vi "Main.vi"() -> ()   [LabVIEW 2012]
uses:
  <vilib>/Platform/TimedLoop/XDataNode/timing_clust.ctl
  <vilib>/Platform/TimedLoop/XDataNode/nitl_modes.ctl
  <vilib>/Platform/TimedLoop/XDataNode/wakeup.ctl
  Sensors and Mapping/Global_grid settings.vi
  <vilib>/FPGAPlugInAG/sbRIO-9636/niLvFpga_Open_sbRIO-9636.vi
  <vilib>/rvi/interface/common/dynamic/niFpgaDynamicAddResources.vi
  <vilib>/Utility/error.llb/Error Cluster From Error Code.vi
  <vilib>/rvi/errors/niLvFpgaAdjustHostInterfaceError.vi
  <vilib>/Analysis/coordinate.llb/2D Cartesian Coordinate Rotation (Scalar).vi
  <vilib>/FPGAPlugInAG/Dynamic/niLvFpga_Close_Dynamic.vi
  <vilib>/Platform/TimedLoop/XDataNode/XDataNode.xnode
  <vilib>/rvi/interface/nirviOpenFPGA/nirviOpenFPGA.xnode
  FPGA Bitfiles/NIARCDemo-kyle_FPGATarget_FPGAToplevel_9c4As6+H2cU.lvbitx
  <vilib>/rvi/interface/nirviReadWriteControl/nirviReadWriteControl.xnode
  <vilib>/robotics/Navigation/shared/WorldMap/OccupancyGridWorldMap/NI_Robotics_OccupancyGridWorldMap.lvclass
  <vilib>/rvi/interface/nirviCloseFPGA/nirviCloseFPGA.xnode
  <vilib>/Platform/TimedLoop/XDataNode/XDNodeRunTimeDep.lvlib
  Compass/Compass IO.lvlib
  Mouse IO/Mouse IO.lvlib
  <vilib>/Analysis/NI_AALPro.lvlib
  NiFpgaLv.dll
  <vilib>/rvi/interface/Simulation/niFpgaSimulationCallBeginRW.vi
panel:
  in  "Max Distance":dbl=0.8
  in  "Robot Velocities":T1 {"Angular Velocity (rad/s)" min=-1.0 max=1.0 scale=1.0..-1.0; "Y Velocity (m/s)" min=-1.0 max=1.0 scale=-1.0..1.0; "X Velocity (m/s)" min=-1.0 max=1.0 scale=-1.0..1.0}
  in  "Enable":bool
  out "Robot Location":cluster{"X array":dbl[], "Y array":dbl[]}(graph)
  out "Robot y":dbl
  out "Robot x":dbl
  out "Heading (deg)":dbl
  out "Object Array":cluster{"Sensor X":dbl, "Sensor Y":dbl}[](array[cluster])
  out "Sensor Distances":fxp<+/-,26,5>[](array[numeric])
  out "Iteration Duration":i64
  out "Sensor position Global":cluster{"Object X":dbl, "Object Y":dbl}
  in  "Robot position Global":T2 {"Orientation (rad)" step=0.1}
  out "Finished late":bool
  out "Object Map":dbl[][](graph)
  in  "x start":i32
  in  "y start":i32
  in  "stop":bool
  # "Goal"
  # "Start"
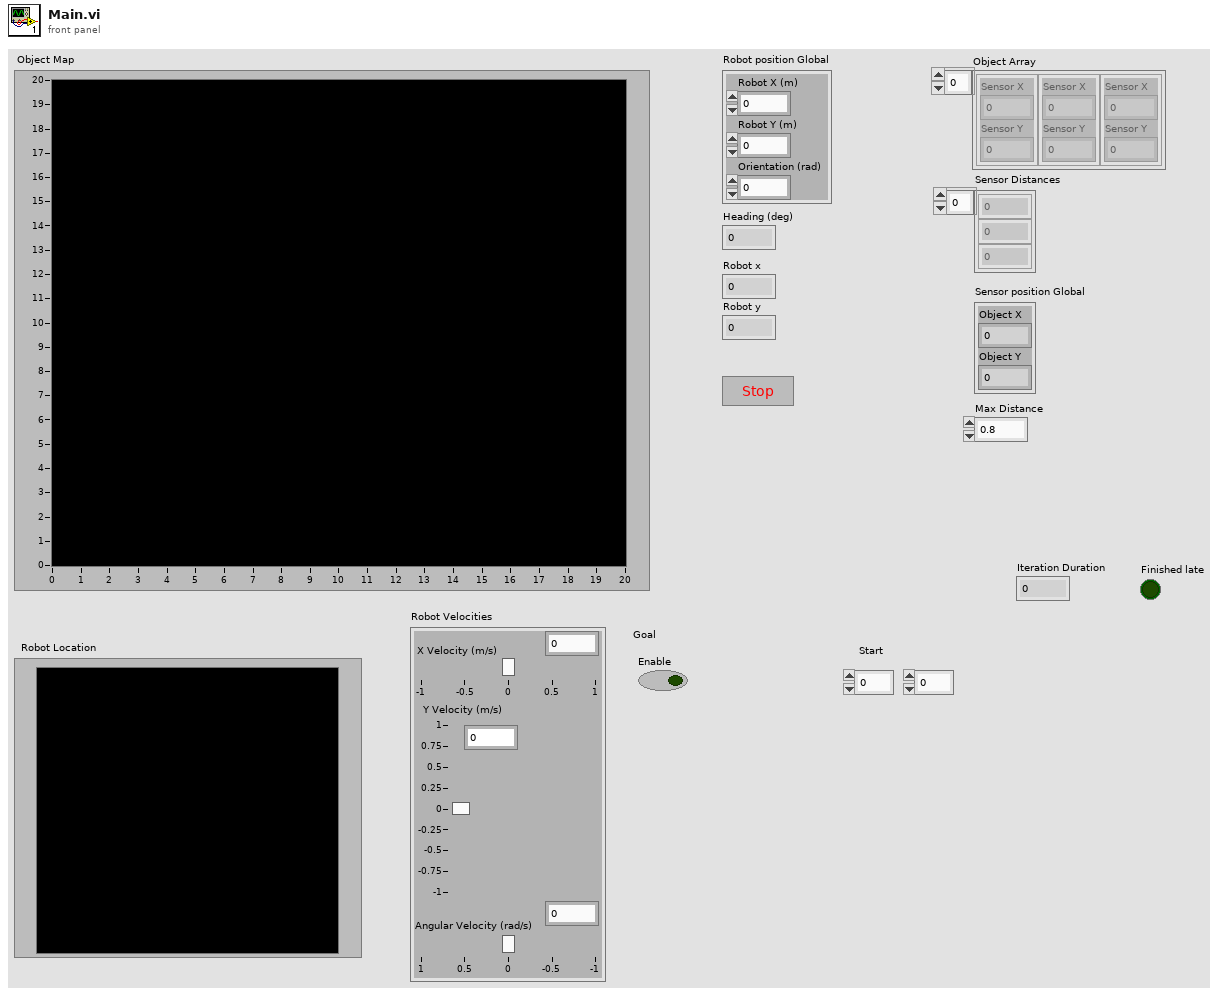
[diagram p1: front panel]
types:
  T1 = cluster{"X Velocity (m/s)":dbl, "Y Velocity (m/s)":dbl, "Angular Velocity (rad/s)":dbl}
  T2 = cluster{"Robot X (m)":dbl, "Robot Y (m)":dbl, "Orientation (rad)":dbl}
  T3 = cluster{"sensor x":dbl, "sensor y":dbl, "sensor rot (rad)":dbl}[]
  T4 = cluster{"X cells":i32, "Y cells":i32, "X size (m)":dbl, "Y size (m)":dbl}
  T5 = cluster{"FPGA VI Reference":refnum<k20>, "Timeout":i32}
  T6 = cluster{"FPGA VI Reference":refnum<k20>, "Port Number":u8}
  T7 = typedef "XDNodeRunTimeDep.lvlib/timing_clust.ctl" = cluster{"Expected End [f-1]":u64, "Actual End [f-1]":u64, "Finished Late? [f-1]":bool, "Expected End [i-1]":u64, "Actual End [i-1]":u64, "Finished Late? [i-1]":bool, "Expected Start [i]":u64, "Actual Start [i]":u64, "Expected Start [f]":u64, "Actual Start [f]":u64, "Source Name":string, "Structure Name":string, "Period":i64, "Deadline":i64, "Offset":i64, "Start":i64, "Priority":i32, "Timeout":i32, "Mode":T8, "Wakeup Reason":T9, "Error":errorcluster, "Source Type":string, "Secondary Source Type":string, "Global End Time":u64, "Global Start Time":u64, "Frame Duration":u64, "Iteration Duration":u64, "Assigned CPU":i32, "I/O Scan Engine Mode":u32}
  T8 = typedef "XDNodeRunTimeDep.lvlib/nitl_modes.ctl" = enum32{"No Change", "Process missed periods, maintain original phase", "Discard missed periods, maintain original phase", "Process missed periods, ignore original phase", "Discard missed periods, ignore original phase"}
  T9 = typedef "XDNodeRunTimeDep.lvlib/wakeup.ctl" = enum32{"Normal", "Aborted", "Asynchronous wakeup", "Timing source error", "Timed loop error", "Timeout"}
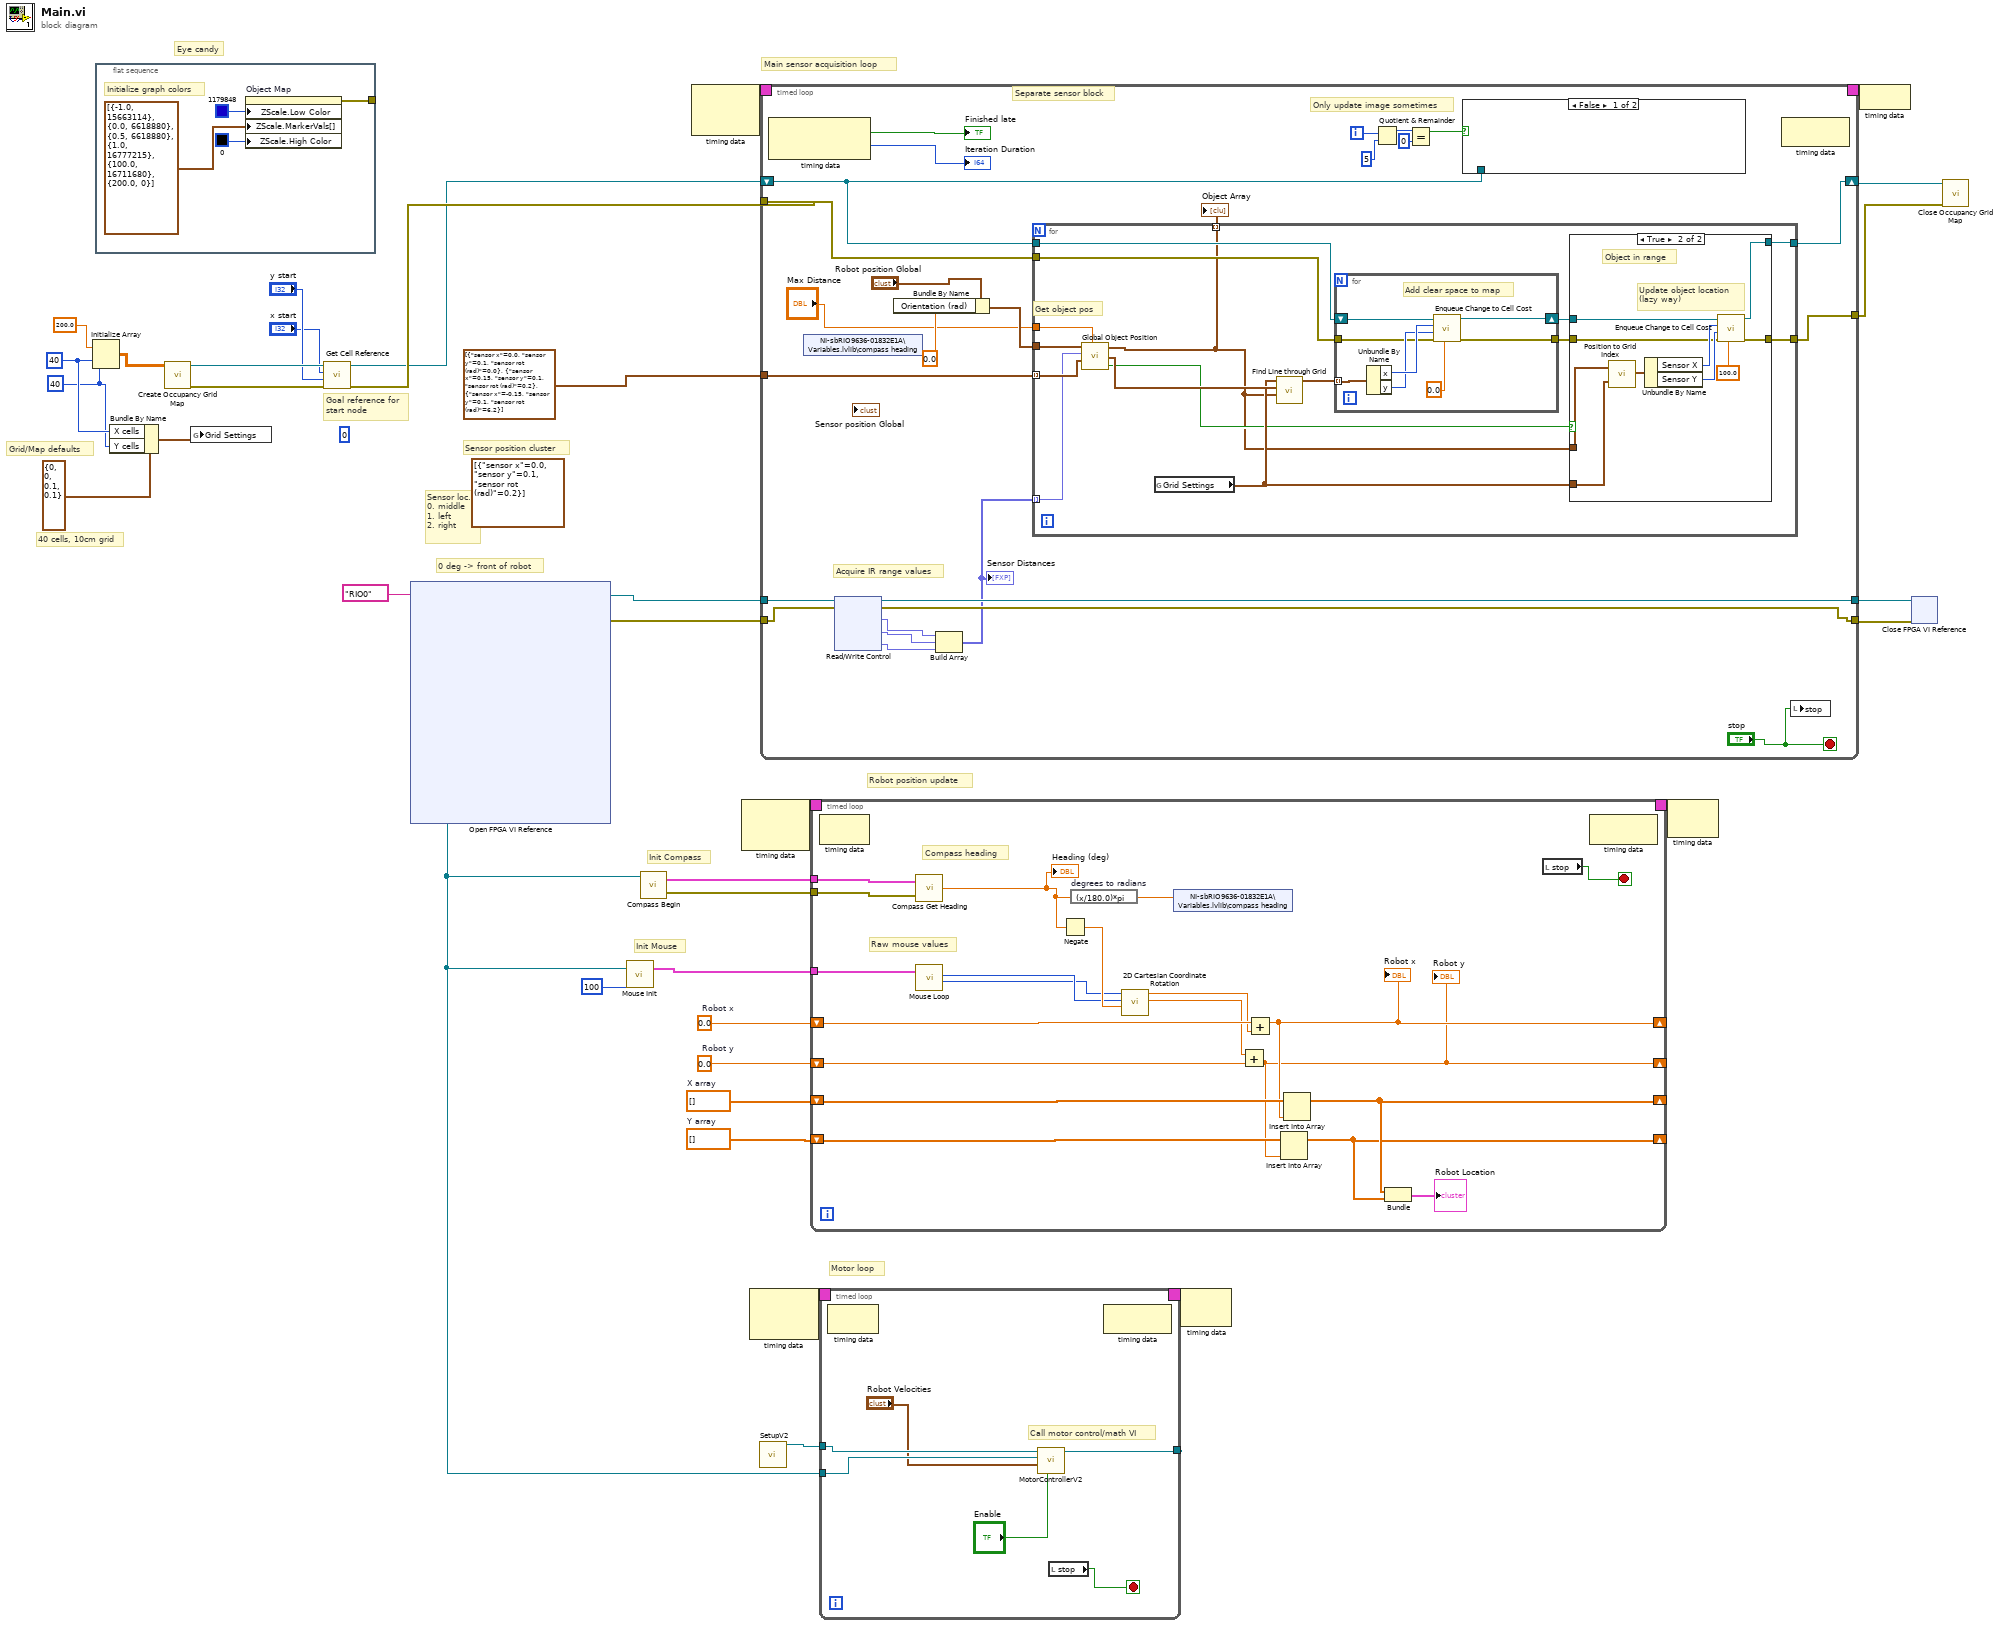
[diagram p0: block diagram]
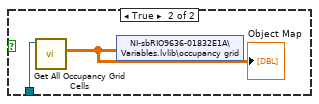
[diagram p3: hidden frame]
diagram:
  w5 = dbl[] []  # Y array
  w6 = dbl[] []  # X array
  w9 = 0.0  # Robot y
  w10 = 0.0  # Robot x
  (unwired) T3 [{"sensor x"=0.0, "sensor y"=0.1, "sensor rot (rad)"=0.0}, {"sensor x"=0.15, "sensor y"=0.1, "sensor rot (rad)"=0.2}, {"sensor x"=-0.15, "sensor y"=0.1, "sensor rot (rad)"=6.2}]
  (unwired) T3 [{"sensor x"=0.0, "sensor y"=0.1, "sensor rot (rad)"=0.2}]
  w24 = 40 ("dimension size")
  w25 = 40 ("dimension size")
  (unwired) 0
  # "Motor loop"
  # "Init Mouse"
  # "Init Compass"
  # "Robot position update"
  # "Main sensor acquisition loop"
  # "Sensor loc.:\n0. middle\n1. left\n2. right"
  # "Sensor position cluster"
  # "Eye candy"
  # "40 cells, 10cm grid"
  # "Grid/Map defaults"
  # "0 deg -> front of robot"
  # "Separate sensor block"
  # "Goal reference for\nstart node"
  n1 = Initialize Array(200.0 ("element"), w25, w24) -> (w29:dbl[][])
  n2 = flat-sequence {
    tunnel: [w36] -> _
    frame #0 {
      # "Initialize graph colors"
      n3 = property on="Object Map" class="IntGraph (strict)"("ZScale.Low Color"=u32 1179848, "ZScale.MarkerVals[]"=cluster{dbl, u32}[] [{-1.0, 15663114}, {0.0, 6618880}, {0.5, 6618880}, {1.0, 16777215}, {100.0, 16711680}, {200.0, 0}], "ZScale.High Color"=u32 0) -> (error out=w36:errorcluster)  [unwired: 2 in, 1 out]
    }
  }
  n4 = Bundle By Name(cluster=T4 {"X cells"=0, "Y cells"=0, "X size (m)"=0.1, "Y size (m)"=0.1} ("Grid Settings"), "X cells"=w25, "Y cells"=w24) -> (w27:T4)
  n5 = call <vilib>:"Create Occupancy Grid Map.vi"("occupancy grid"=w29) -> ("error out"=w32:errorcluster, "map reference out"=w33:refnum<data-value>)  [unwired: 9 in]
  n6 = global write "Global_grid settings.vi" "Grid Settings"(w27) -> ()
  n7 = call <vilib>:"Get Cell Reference.vi"("error in (no error)"=w32, "y"="y start", "x"="x start", "map reference in"=w33) -> ("error out"=w23:errorcluster, "map reference out"=w16:refnum<data-value>)  [unwired: 4 in, 2 out]
  n8 = xnode "Open FPGA VI Reference"("resource name"=tag "RIO0") -> ("FPGA VI Reference Out"=w1:refnum<k20>, "error out"=w20:errorcluster)  [unwired: 1 in]
  n9 = call "Mouse Init.vi"("Timeout (ms)"=100, "FPGA VI Reference In"=w1) -> ("Mouse Sensor"=w11:T5)  [unwired: 1 out]
  n10 = call "Compass Begin.vi"("FPGA VI Reference"=w1) -> ("error out"=w7:errorcluster, "FPGA Information Out"=w8:T6)  [unwired: 3 in]
  n11 = node-c288() -> (w35:T7)  [unwired: 2 in]
  n12 = node-c288() -> (w13:T7)  [unwired: 2 in]
  n13 = node-c288() -> (w4:T7)  [unwired: 2 in]
  n14 = call "SetupV2.vi"() -> ("mecanum steering frame out"=w2:refnum<class "NI_Robotics_Mecanum Steering Frame.lvclass">)  [unwired: 10 in, 1 out]
  n15 = timed-loop {
    timing: w35 -> [_]
    timing-out: [_] -> w34
    shift-right: [w58] -> w22
    shift-left: w16 -> [w51]
    tunnel: [w57] -> w21
    tunnel: w23 -> [w56]
    tunnel: T3 [{"sensor x"=0.0, "sensor y"=0.1, "sensor rot (rad)"=0.0}, {"sensor x"=-0.15, "sensor y"=0.1, "sensor rot (rad)"=0.0872664625997165}, {"sensor x"=0.15, "sensor y"=0.1, "sensor rot (rad)"=6.19591884457987}] -> [w47]
    tunnel: [w49] -> w19
    tunnel: w1 -> [w55]
    tunnel: [w48] -> w18
    tunnel: w20 -> [w54]
    i -> [w63]
    stop <- "stop" stop-if-true
    # "Acquire IR range values"
    # "Only update image sometimes"
    n16 = node-c288() -> (→"Finished late":bool, →"Iteration Duration":i64)  [unwired: 1 in]
    n17 = shared-variable "NI-sbRIO9636-01832E1A\\Variables.lvlib\\compass heading"() -> ()  [unwired: 1 in, 2 out]
    n18 = xnode "Read/Write Control"("FPGA VI Reference In"=w55, "error in"=w54) -> ("FPGA VI Reference Out"=w49:refnum<k20>, "error out"=w48:errorcluster, "IR 0"=w53:fxp<+/-,24,5>, "IR 2"=w50:fxp<+/-,24,5>, "IR 3"=w52:fxp<+/-,24,5>)
    n19 = Bundle By Name(cluster="Robot position Global", "Orientation (rad)"=0.0 ("compass heading")) -> (w42:T2)
    n20 = Build Array(w53, w50, w52) -> (w46:fxp<+/-,24,5>[])
    "Sensor Distances" <- w46
    n21 = for {
      tunnel: w42 -> [w80]
      tunnel: [w79] -> w58
      tunnel: [w78] -> w57
      tunnel: w56 -> [w77]
      tunnel: "Max Distance" -> [w76]
      tunnel: w51 -> [w74]
      tunnel: w47 -> [w68] mode=indexing
      tunnel: w46 -> [w67] mode=indexing
      tunnel: [w66] -> w45 mode=indexing
      # "Get object pos"
      n22 = call "Global Object Position.vi"("Robot position Global"=w80, "Distance (m)"=w67, "Sensor Position"=w68, "Max Distance"=w76) -> ("Object position Global"=w66:cluster{"Sensor X":dbl, "Sensor Y":dbl}, "Sensor position Global"=w75:cluster{"Object X":dbl, "Object Y":dbl}, "In Range?"=w69:bool)  [unwired: 1 in]
      n23 = global read "Global_grid settings.vi" "Grid Settings"() -> (w73:T4)
      n24 = call "Find Line through Grid.vi"("Point 2"=w66, "Point 1"=w75, "Grid Settings"=w73) -> ("Array"=w72:cluster{"x":i32, "y":i32}[])  [unwired: 8 in]
      n25 = for {
        tunnel: w72 -> [w100] mode=indexing
        shift-right: [w98] -> w71
        shift-left: w74 -> [w99]
        tunnel: [w94] -> w70
        tunnel: w77 -> [w93]
        # "Add clear space to map"
        n26 = Unbundle By Name(w100) -> ("x"=w97:i32, "y"=w96:i32)
        n27 = call <vilib>:"Enqueue Change to Cell Cost.vi"("cost"=0.0, "error in (no error)"=w93, "y"=w96, "x"=w97, "map reference in"=w99) -> ("error out"=w94:errorcluster, "map reference out"=w98:refnum<data-value>)  [unwired: 5 in]
      }
      n28 = case shown="True" w69 {
        tunnel: [w82 w92] -> w79
        tunnel: w66 -> [_ w91]
        tunnel: w73 -> [_ w90]
        tunnel: [w81 w89] -> w78
        tunnel: w71 -> [w82 w88]
        tunnel: w70 -> [w81 w83]
        frame False {
          # "No oject in range"
        }
        frame True {
          # "Object in range"
          # "Update object location\n(lazy way)"
          n29 = call "Position to Grid Index.vi"("Grid Settings"=w90, "Global Position"=w91) -> ("Grid Index"=w86:cluster{"Sensor X":i32, "Sensor Y":i32})  [unwired: 1 out]
          n30 = Unbundle By Name(w86) -> ("Sensor X"=w85:i32, "Sensor Y"=w84:i32)
          n31 = call <vilib>:"Enqueue Change to Cell Cost.vi"("cost"=100.0, "error in (no error)"=w83, "y"=w84, "x"=w85, "map reference in"=w88) -> ("error out"=w89:errorcluster, "map reference out"=w92:refnum<data-value>)  [unwired: 5 in]
        }
      }
    }
    "Object Array" <- w45
    n32 = Quotient & Remainder(x=w63, y=5) -> (x-y*floor(x/y)=w62:i32)  [unwired: 1 out]
    n33 = Equal?(x=w62, y=0) -> (x = y?=w60:bool)
    n34 = case shown="False" w60 {
      tunnel: w51 -> [_ w102]
      frame False {
      }
      frame True {
        n35 = call <vilib>:"Get All Occupancy Grid Cells.vi"("map reference in"=w102) -> ("occupancy grid"=w101:dbl[][])  [unwired: 8 in, 2 out]
        "Object Map" <- w101
        n36 = shared-variable "NI-sbRIO9636-01832E1A\\Variables.lvlib\\occupancy grid"(w101) -> ()  [unwired: 1 in, 1 out]
      }
    }
    n37 = node-c288() -> ()  [unwired: 1 in, 1 out]
    n38 = local write "stop"("stop") -> ()
  }
  n39 = timed-loop {
    timing: w13 -> [_]
    timing-out: [_] -> w12
    tunnel: w11 -> [w126]
    shift-right: [w110] -> _
    shift-left: w10 -> [w122]
    shift-right: [w109] -> _
    shift-left: w9 -> [w121]
    tunnel: w8 -> [w125]
    tunnel: w7 -> [w124]
    shift-right: [w111] -> _
    shift-left: w5 -> [w113]
    shift-right: [w112] -> _
    shift-left: w6 -> [w114]
    stop <- w116 stop-if-true
    # "Compass heading"
    # "Raw mouse values"
    n40 = node-c288() -> ()  [unwired: 1 in, 1 out]
    n41 = call "Compass Get Heading.vi"("FPGA Information In"=w125, "error in (no error)"=w124) -> ("Heading (deg)"=w108:dbl)  [unwired: 2 out]
    "Heading (deg)" <- w108
    n42 = call "Mouse Loop.vi"("Mouse Sensor In"=w126) -> ("x displacement"=w118:i8, "y displacement"=w117:i8)  [unwired: 2 in, 1 out]
    n43 = Negate(x=w108) -> (-x=w123:dbl)
    n44 = expression code="(x/180.0)*pi" "degrees to radians"(w108) -> (w107:dbl)
    n45 = call-poly <vilib>:"2D Cartesian Coordinate Rotation.vi"("theta"=w123, "y"=w118, "x"=w117) -> ("y out"=w119:dbl, "x out"=w120:dbl)  [unwired: 6 in, 1 out]
    n46 = shared-variable "NI-sbRIO9636-01832E1A\\Variables.lvlib\\compass heading"(w107) -> ()  [unwired: 1 in, 1 out]
    n47 = Add(x=w119, y=w121) -> (x+y=w109:dbl)
    "Robot y" <- w109
    n48 = Add(x=w122, y=w120) -> (x+y=w110:dbl)
    "Robot x" <- w110
    n49 = Insert Into Array(array=w113, new element=w109) -> (w111:dbl[])  [unwired: 1 in]
    n50 = Insert Into Array(array=w114, new element=w110) -> (w112:dbl[])  [unwired: 1 in]
    n51 = Bundle("X array"=w112, "Y array"=w111) -> (→"Robot Location":cluster{"X array":dbl[], "Y array":dbl[]})  [unwired: 1 in]
    n52 = local read "stop"() -> (w116:bool)
    n53 = node-c288() -> ()  [unwired: 1 in, 1 out]
  }
  n54 = timed-loop {
    timing: w4 -> [_]
    timing-out: [_] -> w3
    tunnel: w2 -> [w134]
    tunnel: w1 -> [w132]
    tunnel: [w130] -> _
    stop <- w129 stop-if-true
    # "Call motor control/math VI"
    n55 = node-c288() -> ()  [unwired: 1 in, 1 out]
    n56 = call "MotorControllerV2.vi"("Enable"="Enable", "Robot Velocities"="Robot Velocities", "FPGA VI Reference In"=w132, "mecanum steering frame in"=w134) -> ("steering frame out"=w130:refnum<class "NI_Robotics_Mecanum Steering Frame.lvclass">)  [unwired: 6 in, 1 out]
    n57 = local read "stop"() -> (w129:bool)
    n58 = node-c288() -> ()  [unwired: 1 in, 1 out]
  }
  n59 = node-c288(w3) -> ()  [unwired: 1 out]
  n60 = node-c288(w12) -> ()  [unwired: 1 out]
  n61 = node-c288(w34) -> ()
  n62 = xnode "Close FPGA VI Reference"("FPGA VI Reference In"=w19, "error in"=w18) -> ()  [unwired: 1 out]
  n63 = call <vilib>:"Close Occupancy Grid Map.vi"("error in (no error)"=w21, "map reference in"=w22) -> ()  [unwired: 9 in, 1 out]
